vi "Read ESI Files on Host PC.vi"(8 "error in (no error)":errorcluster) -> (0 "error out":errorcluster, 3 "Existing Host Profiles":string[](array[string]))   [LabVIEW 2020, in "SEECD System Explorer.lvlib"]
uses:
  SEECD System Explorer.lvlib
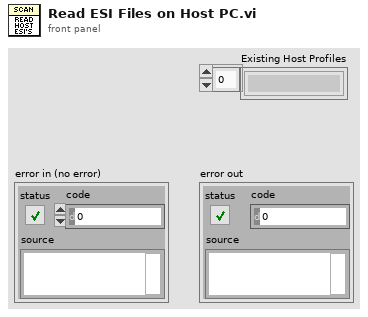
[diagram p1: front panel]
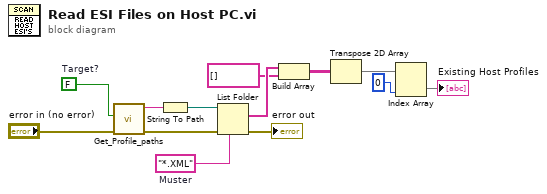
[diagram p0: block diagram]
diagram:
  w1 = FALSE  # Target?
  w3 = "*.XML"  # Muster
  n1 = call "Get_Profile_paths.vi"("error in (no error)"="error in (no error)", "Target?"=w1) -> ("error out"=w6:errorcluster, "profileDestPath"=w5:string)  [unwired: 8 in]
  n2 = String To Path(string=w5) -> (path=w4:path)
  n3 = List Folder(path=w4, pattern=w3, error in=w6) -> (filenames=w10:string[], error out=→"error out":errorcluster)  [unwired: 1 in, 2 out]
  n4 = Build Array(w10, string[] [] ("Element")) -> (w8:string[][])
  n5 = Transpose 2D Array(2D array=w8) -> (transposed array=w11:string[][])
  n6 = Index Array(array=w11, index (col)=0) -> (element=→"Existing Host Profiles":string[])  [unwired: 1 in]
